vi "test property.vi"() -> ()   [LabVIEW 2017]
uses:
  Routines.ctl
  Starting Position.ctl
panel:
  out "Strings [] 2":string[](array[string])
  out "Strings []":string[](array[string])
  in  "Starting Position":T1
  in  "Routines":T2
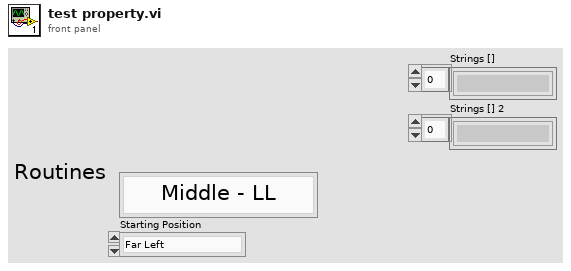
[diagram p1: front panel]
types:
  T1 = typedef "Starting Position.ctl" = enum16{"Far Left", "Middle", "Far Right"}
  T2 = typedef "Routines.ctl" = enum16{"Middle - LL", "Middle - LR", "Middle - RL", "Middle - RR", "Far Right - LL", "Far Right - LR", "Far Right - RL", "Far Right - RR", "Far Left - LL", "Far Left - LR", "Far Left - RL", "Far Left - RR"}
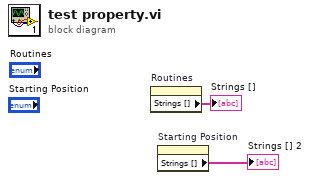
[diagram p0: block diagram]
diagram:
  n1 = property on="Routines" class="Enum (strict)"() -> ("Strings []"=→"Strings []":string[])  [unwired: 2 in, 2 out]
  n2 = property on="Starting Position" class="Enum (strict)"() -> ("Strings []"=→"Strings [] 2":string[])  [unwired: 2 in, 2 out]
